vi "integration_test_for_main.vi"() -> ()   [LabVIEW 2019]
uses:
  <instrlib>/Yokogawa WT200 Series/Yokogawa WT200 Series.lvlib
panel:
  in  "stop":bool
  out "output cluster":T1
  out "Waveform Chart 2":cluster{sgl, sgl, sgl, sgl}(graph)
  out "Waveform Chart":cluster{sgl, sgl, sgl, sgl}(graph)
  out "Measure Values":sgl[](array[numeric]) format="%^.3e"
  in  "Second (0)":u32 max=59 step=1
  in  "error in (no error)":errorcluster
  in  "VISA resource name":refnum<visa-resource-name>
  in  "Minute (0)":u32 max=59 step=1
  in  "Hour (0)":u32 max=10000
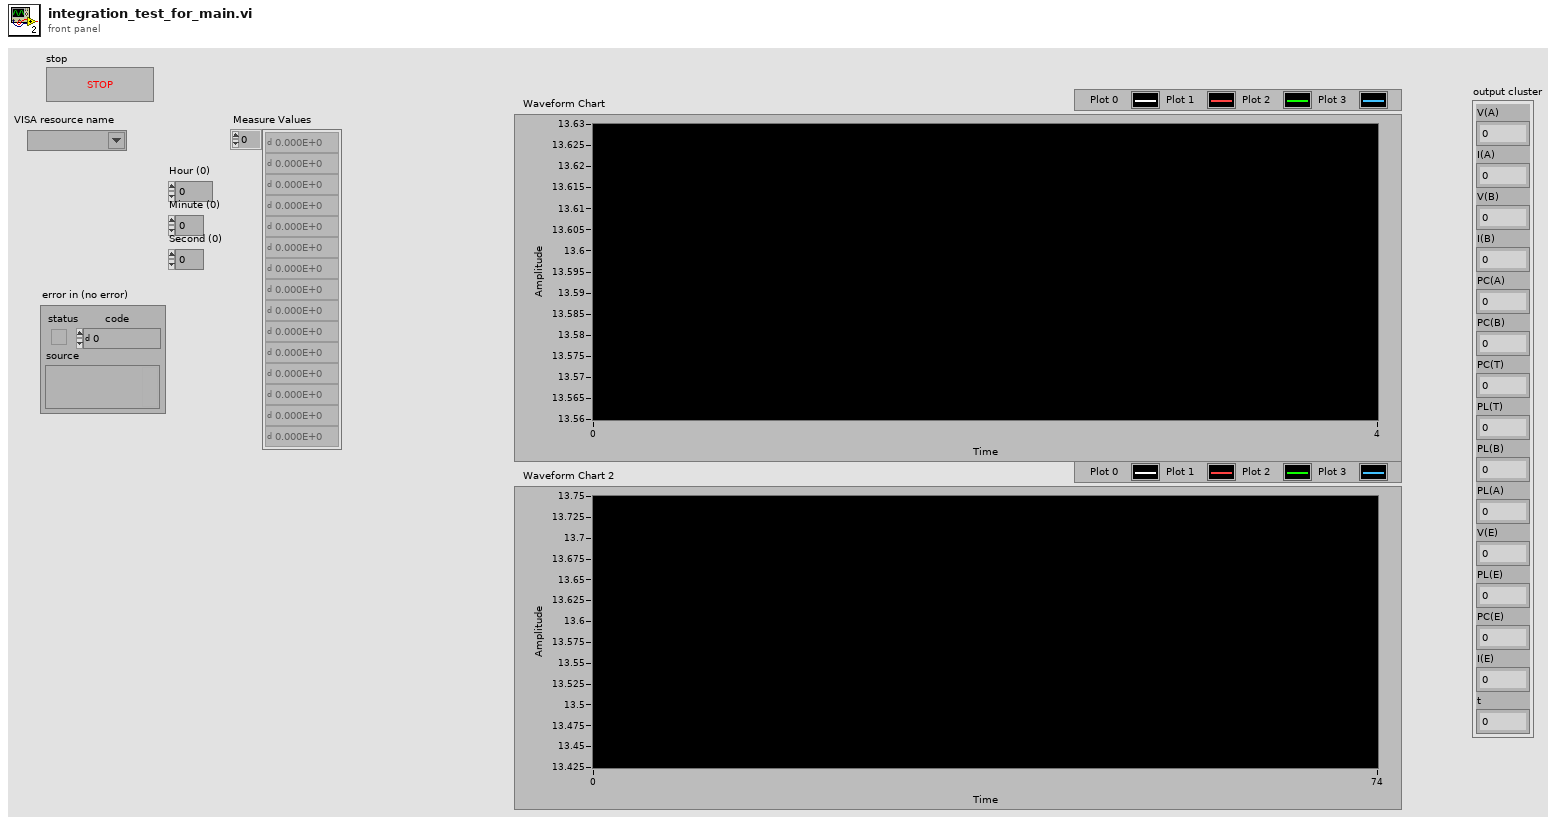
[diagram p1: front panel]
types:
  T1 = cluster{"V(A)":dbl, "I(A)":dbl, "V(B)":dbl, "I(B)":dbl, "PC(A)":dbl, "PC(B)":dbl, "PC(T)":dbl, "PL(T)":dbl, "PL(B)":dbl, "PL(A)":dbl, "V(E)":dbl, "PL(E)":dbl, "PC(E)":dbl, "I(E)":dbl, "t":dbl}
  T2 = cluster{"PI(A)":sgl, "PI(B)":sgl, "PI(T)":sgl, "PI(E)":sgl}
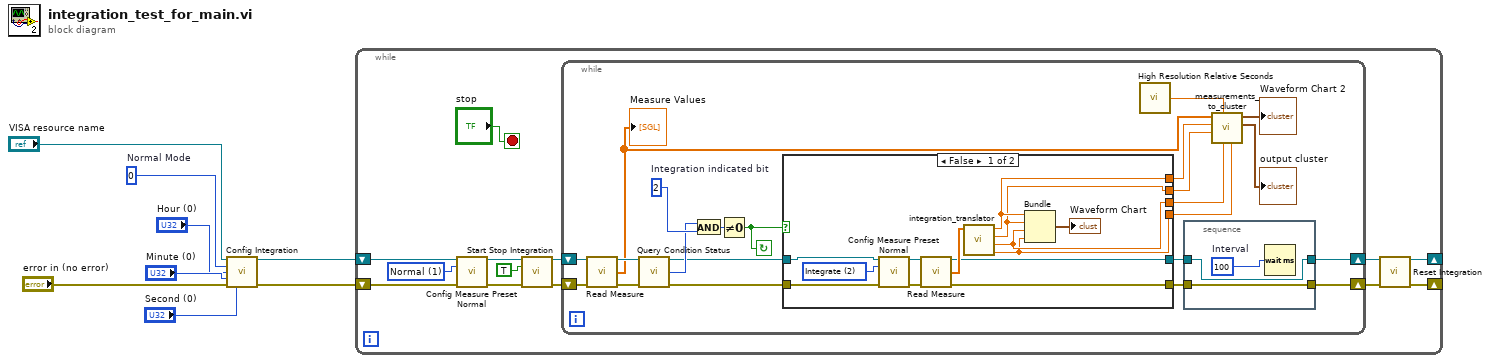
[diagram p0: block diagram]
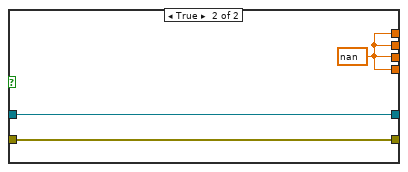
[diagram p2: hidden frame]
diagram:
  w1 = u16 0  # Normal Mode
  n1 = call <instrlib>:"Config Integration.vi"("VISA resource name"="VISA resource name", "Integ Mode (0: Normal)"=w1, "Hour (0)"="Hour (0)", "Minute (0)"="Minute (0)", "error in (no error)"="error in (no error)", "Second (0)"="Second (0)") -> ("VISA resource name out"=w8:refnum<visa-resource-name>, "error out"=w7:errorcluster)  [unwired: 8 in]
  n2 = while {
    shift-right: [w11] -> _
    shift-left: w8 -> [w21]
    shift-right: [w10] -> _
    shift-left: w7 -> [w20]
    stop <- "stop" stop-if-true
    w14 = u16 1 items=["Clear", "Normal", "Integrate"] ("Preset Pattern (0: Clear)")
    n3 = call <instrlib>:"Config Measure Preset Normal.vi"("VISA resource name"=w21, "Preset Pattern (0: Clear)"=w14, "error in (no error)"=w20) -> ("VISA resource name out"=w16:refnum<visa-resource-name>, "error out"=w15:errorcluster)  [unwired: 11 in]
    n4 = call <instrlib>:"Start Stop Integration.vi"("VISA resource name"=w16, "Start/Stop (F: Stop)"=TRUE, "error in (no error)"=w15) -> ("VISA resource name out"=w19:refnum<visa-resource-name>, "error out"=w18:errorcluster)  [unwired: 11 in]
    n5 = while {
      shift-left: w19 -> [w40]
      shift-right: [w26] -> w12
      shift-left: w18 -> [w37]
      shift-right: [w24] -> w9
      stop <- w36 continue-if-true
      w43 = u16 2  # Integration indicated bit
      n6 = call <instrlib>:"Read Measure.vi"("VISA resource name"=w40, "error in (no error)"=w37) -> ("VISA resource name out"=w39:refnum<visa-resource-name>, "Measure Value"=w30:sgl[], "error out"=w38:errorcluster)  [unwired: 10 in, 1 out]
      "Measure Values" <- w30
      n7 = call <instrlib>:"Query Condition Status.vi"("VISA resource name"=w39, "error in (no error)"=w38) -> ("VISA resource name out"=w23:refnum<visa-resource-name>, "Condition"=w41:u16, "error out"=w22:errorcluster)  [unwired: 11 in]
      n8 = And(x=w41, y=w43) -> (x .and. y?=w42:u16)
      n9 = Not Equal To 0?(x=w42) -> (x != 0?=w36:bool)
      n10 = case shown="False" w36 {
        tunnel: [w54 w62] -> w35
        tunnel: [w53 w62] -> w34
        tunnel: [w52 w62] -> w33
        tunnel: [w51 w62] -> w32
        tunnel: [w50 w61] -> w27
        tunnel: [w49 w60] -> w25
        tunnel: w23 -> [w48 w61]
        tunnel: w22 -> [w47 w60]
        frame False {
          w56 = u16 2 items=["Clear", "Normal", "Integrate"] ("Preset Pattern (0: Clear)")
          n11 = call <instrlib>:"Config Measure Preset Normal.vi"("VISA resource name"=w48, "Preset Pattern (0: Clear)"=w56, "error in (no error)"=w47) -> ("VISA resource name out"=w59:refnum<visa-resource-name>, "error out"=w58:errorcluster)  [unwired: 11 in]
          n12 = call <instrlib>:"Read Measure.vi"("VISA resource name"=w59, "error in (no error)"=w58) -> ("VISA resource name out"=w50:refnum<visa-resource-name>, "Measure Value"=w57:sgl[], "error out"=w49:errorcluster)  [unwired: 10 in, 1 out]
          n13 = call "integration_translator.vi"("Valores integração"=w57) -> ("PI(E)"=w51:sgl, "PI(T)"=w52:sgl, "PI(B)"=w53:sgl, "PI(A)"=w54:sgl)  [unwired: 7 in]
          n14 = Bundle("PI(A)"=w54, "PI(B)"=w53, "PI(T)"=w52, "PI(E)"=w51) -> (→"Waveform Chart":T2)  [unwired: 1 in]
        }
        frame True {
          w62 = nan
        }
      }
      n15 = call <vilib>:"High Resolution Relative Seconds.vi"() -> ("relative seconds"=w31:dbl)
      n16 = stacked-sequence {
        tunnel: w27 -> [w45]
        tunnel: [w45] -> w26
        tunnel: w25 -> [w44]
        tunnel: [w44] -> w24
        frame #0 {
          w46 = u32 100  # Interval
          n17 = Wait (ms)(milliseconds to wait=w46) -> ()  [unwired: 1 out]
        }
      }
      n18 = call "measurements_to_cluster.vi"("PI(E)"=w32, "PI(T)"=w33, "relative seconds"=w31, "PI(B)"=w34, "PI(A)"=w35, "Measure Value"=w30) -> ("watt cluster"=→"output cluster":T1, "chart out"=→"Waveform Chart 2":cluster{sgl, sgl, sgl, sgl})  [unwired: 4 in]
    }
    n19 = call <instrlib>:"Reset Integration.vi"("VISA resource name"=w12, "error in (no error)"=w9) -> ("VISA resource name out"=w11:refnum<visa-resource-name>, "error out"=w10:errorcluster)  [unwired: 12 in]
  }
